vi "set value DBL.vi"(8 "error in (no error)":errorcluster, 10 "Payload":cluster{"name":string, "value":dbl}, 11 "VI Ref":refnum<vi>) -> (0 "error out":errorcluster, 3 "return value":string)   [LabVIEW 2020, in "ui-testing.lvlib"]
uses:
  ui-testing.lvlib
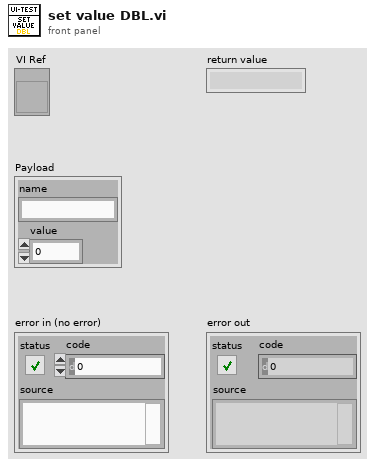
[diagram p1: front panel]
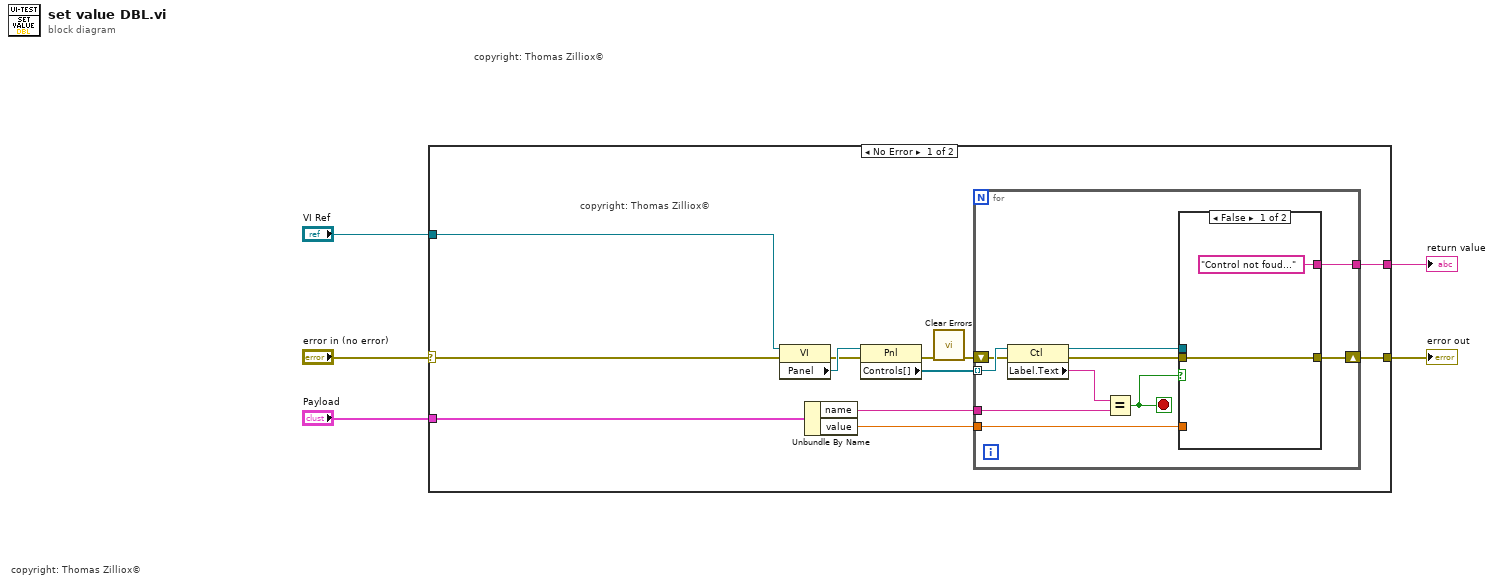
[diagram p0: block diagram]
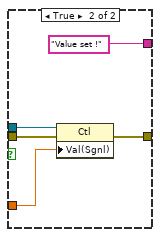
[diagram p2: hidden frame]
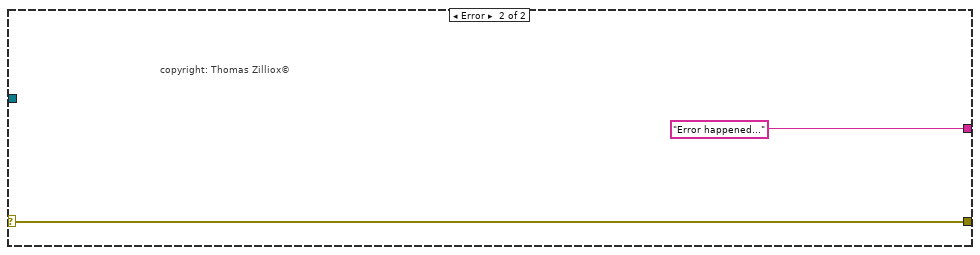
[diagram p3: hidden frame]
diagram:
  # "copyright: Thomas Zilliox©"
  # "copyright: Thomas Zilliox©"
  n1 = case shown="No Error" "error in (no error)" {
    selector: "error in (no error)" -> [w11 w36]
    tunnel: [w8 w36] -> w4
    tunnel: [w9 "Error happened..."] -> w3
    tunnel: "VI Ref" -> [w7 _]
    tunnel: "Payload" -> [w6 _]
    frame No Error {
      # "copyright: Thomas Zilliox©"
      n2 = property class="VI"(reference=w7, error in=w11) -> (error out=w15:errorcluster, "Panel"=w17:refnum<vi>)  [unwired: 1 out]
      n3 = Unbundle By Name(w6) -> ("name"=w13:string, "value"=w12:dbl)
      n4 = property class="Pnl"(reference=w17, error in=w15) -> (error out=w14:errorcluster, "Controls[]"=w16:refnum<vi>[])  [unwired: 1 out]
      n5 = call <vilib>:"Clear Errors.vi"("error in (no error)"=w14) -> ("error out"=w10:errorcluster)  [unwired: 5 in, 1 out]
      n6 = for {
        tunnel: w16 -> [w27] mode=indexing
        tunnel: w13 -> [w25]
        tunnel: w12 -> [w21]
        shift-right: [w19] -> w8
        shift-left: w10 -> [w20]
        tunnel: [w18] -> w9
        stop <- w22 stop-if-true
        n7 = property class="Ctl"(reference=w27, error in=w20) -> (reference out=w23:refnum<vi>, error out=w24:errorcluster, "Label.Text"=w26:string)
        n8 = Equal?(x=w26, y=w25) -> (x = y?=w22:bool)
        n9 = case shown="False" w22 {
          tunnel: w24 -> [w29 w34]
          tunnel: w23 -> [_ w33]
          tunnel: w21 -> [_ w32]
          tunnel: [w29 w31] -> w19
          tunnel: ["Control not foud..." "Value set !"] -> w18
          frame False {
          }
          frame True {
            n10 = property class="Ctl"(reference=w33, error in=w34, "Val(Sgnl)"=w32) -> (error out=w31:errorcluster)  [unwired: 1 out]
          }
        }
      }
    }
    frame Error {
      # "copyright: Thomas Zilliox©"
    }
  }
  "error out" <- w4
  "return value" <- w3
